vi "ReplaceGroup.vi"(8 "error in (no error)":errorcluster, 9 "Selected Grp":T1, 10 "Group Info":refnum<class "ChanGrp.lvclass">, 11 "Chassis Cfg":refnum<class "ChassisCfg.lvclass">) -> (0 "error out":errorcluster, 1 "Selected Grp":T1, 3 "Chassis Cfg":refnum<class "ChassisCfg.lvclass">)   [LabVIEW 2018, in "Configuration Grandmaster.lvlib" / "ChassisCfg.lvclass"]
uses:
  ChassisCfg.lvclass
  Common/Controls/Selected Group.ctl
  Common/Controls/TE_Designator.ctl
  Class Chan Group/ChanGrp.lvclass
  ChassisCfg.lvclass/ChassisCfg.ctl
  Class Timing Group/TimingGrp.lvclass
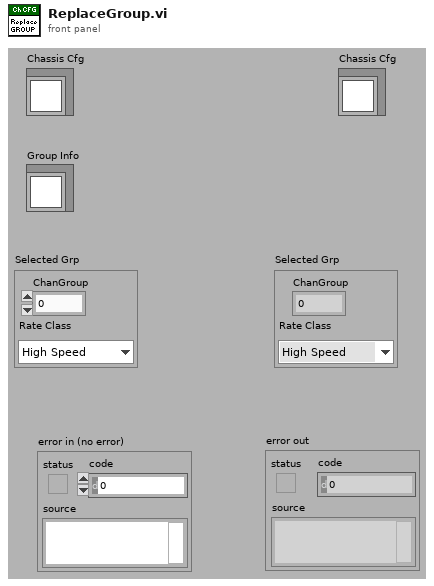
[diagram p1: front panel]
types:
  T1 = typedef "Selected Group.ctl" = cluster{"ChanGroup":i32, "Rate Class":T2}
  T2 = typedef "TE_Designator.ctl" = enum16{"High Speed", "Low Speed"}
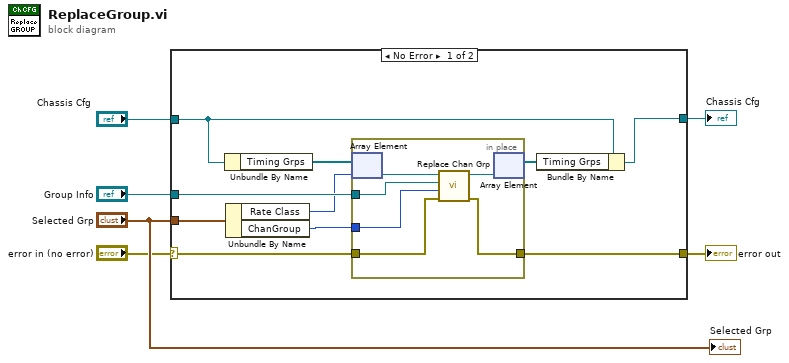
[diagram p0: block diagram]
diagram:
  n1 = case shown="No Error" "error in (no error)" {
    selector: "error in (no error)" -> [w11 w23]
    tunnel: "Selected Grp" -> [w15 _]
    tunnel: "Group Info" -> [w14 _]
    tunnel: "Chassis Cfg" -> [w13 w24]
    tunnel: [w12 w24] -> w3
    tunnel: [w10 w23] -> w1
    frame No Error {
      n2 = Unbundle By Name(w13) -> ("Timing Grps"=w9:refnum<class "TimingGrp.lvclass">[])
      n3 = Unbundle By Name(w15) -> ("Rate Class"=w7:T2, "ChanGroup"=w16:i32)
      n4 = in-place {
        in-place-border: w16 -> [w22]
        in-place-border: w14 -> [w21]
        in-place-border: w11 -> [w20]
        in-place-border: [w19] -> w10
        n5 = in-place-array #1(w9, w7) -> (w18:refnum<class "TimingGrp.lvclass">)
        n6 = call "Replace Chan Grp.vi"("error in (no error)"=w20, "ChanGroupPos"=w22, "ChanGrp to Add"=w21, "TimingGrp in"=w18) -> ("error out"=w19:errorcluster, "TimingGrp out"=w17:refnum<class "TimingGrp.lvclass">)  [unwired: 6 in]
        n7 = in-place-array #1(w17) -> (w8:refnum<class "TimingGrp.lvclass">[])  [unwired: 1 out]
      }
      n8 = Bundle By Name(cluster=w13, "Timing Grps"=w8) -> (w12:refnum<class "ChassisCfg.lvclass">)
    }
    frame Error {
    }
  }
  "Chassis Cfg" <- w3
  "error out" <- w1
  "Selected Grp" <- "Selected Grp"
